vi "Constants.vi"() -> ()   [LabVIEW 2020, in "FlexRay Custom Device Shared.lvlib"]
doc: "Use this Global VI to access the GUIDs assigned to the page resources of the Custom Device."
uses:
  FlexRay Custom Device Shared.lvlib
panel:
  in  "Tab Control":enum32{"GUIDS", "Constants", "Properties"}(tab)
  in  "Delete Multiple Menu":string="07a6682c-c643-4e6b-9fab-aaf67c512cbc"
  in  "POC State Page":string="ec354db5-9c8d-46eb-a3f4-59bfa10bb239"
  in  "Node Page":string="41ebe26f-c608-450f-b619-084b7dff9332"
  in  "Enable_Disable Page":string="ec354db5-9c8d-46eb-a3f4-59bfa10bb237"
  in  "Add Signal Menu":string="a9a10e21-58a4-4b98-aa49-6bc2047028e5"
  in  "Signal Page":string="c15b0c5e-0082-413d-b32b-8504b9b0c532"
  in  "Frame Page":string="58e98b2a-a2de-4811-bb4b-d9c14c05292d"
  in  "Event Page":string="cdaa898b-86df-49d7-a3b3-fd26b020a728"
  in  "Cyclic Page":string="373b1fd3-81ba-4d8e-b3d4-95e0417f15b0"
  in  "Outgoing Page":string="75018574-3c49-443e-8842-0b959c2eb90f"
  in  "Incoming Page":string="c98d7020-8536-4134-a3e2-a734e8e0249f"
  in  "FlexRay Custom Device":string="852c7a30-5944-4e88-8c64-fbd6d2862294"
  in  "Version":string="1.4.1"
  in  "Frame":string="FrameRef"
  in  "Frame ID":string="Frame ID"
  in  "StartUp?":string="Startup?"
  in  "FRFrameType":string="FRFrameType"
  in  "FRSignal":string="FRSignal"
  in  "FRConfig":string="FRConfig"
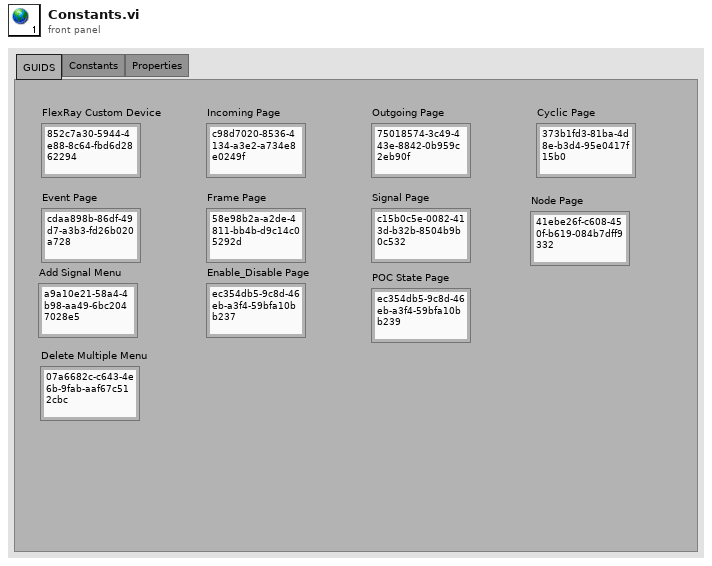
[diagram p1: front panel]
diagram:
